vi "ConnectToAdaptorr02.vi"(1 "error in (no error)":errorcluster) -> (0 "error out":errorcluster, 2 "VISA resource name out":refnum<visa-resource-name>)   [LabVIEW 2011]
uses:
  <vilib>/Utility/error.llb/DialogType.ctl
  <vilib>/Instr/_visa.llb/VISA Configure Serial Port (Instr).vi
panel:
  out "message":string="AdaptTorr error!"
  in  "flow control":u16(ring) items=["None"=0, "XON/XOFF"=1, "RTS/CTS"=2, "DTR/DSR"=4]
  in  "stop bits":u16(ring)=20 items=["2"=10, "1.5"=15, "2.0"=20]
  in  "parity":u16(ring) items=["None", "Odd", "Even", "Mark", "Space"]
  in  "data bits":u16=8 min=5 max=8 step=1
  in  "VISA resource name":refnum<visa-resource-name>="COM8"
  in  "baud rate":u32=9600
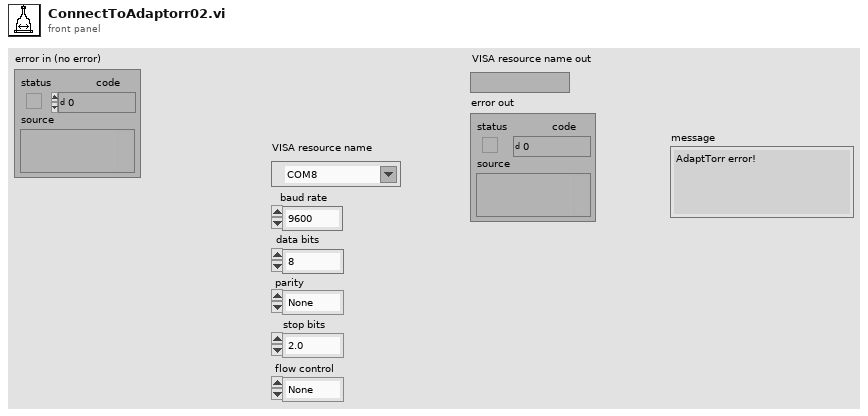
[diagram p1: front panel]
types:
  T1 = typedef "DialogType.ctl" = u16
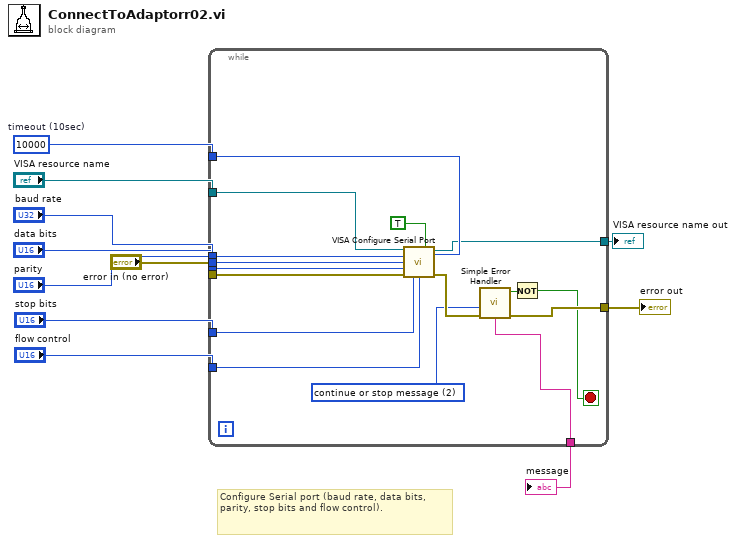
[diagram p0: block diagram]
diagram:
  w8 = u32 10000  # timeout (10sec)
  # "Configure Serial port (baud rate, data bits, parity, stop bits and flow control)."
  n1 = while {
    tunnel: "baud rate" -> [w27]
    tunnel: "VISA resource name" -> [w26]
    tunnel: "parity" -> [w25]
    tunnel: w8 -> [w24]
    tunnel: "stop bits" -> [w23]
    tunnel: "flow control" -> [w22]
    tunnel: "data bits" -> [w21]
    tunnel: [w20] -> w4
    tunnel: "error in (no error)" -> [w19]
    tunnel: [w18] -> w2
    tunnel: [w17] -> w1
    stop <- w16 stop-if-true
    w13 = T1 2 items=["no dialog", "OK message", "continue or stop message", "OK message + warnings", "continue/stop + warnings"] ("type of dialog (OK msg:1)")
    n2 = call-poly "VISA Configure Serial Port"("VISA resource name"=w26, "timeout (10sec)"=w24, "Enable Termination\nChar (T)"=TRUE ("Enable Termination\nChar (T)"), "baud rate (9600)"=w27, "data bits (8)"=w21, "parity (0:none)"=w25, "error in (no error)"=w19, "stop bits (10: 1 bit)"=w23, "flow control (0:none)"=w22) -> ("VISA resource name out"=w20:refnum<visa-resource-name>, "error out"=w14:errorcluster)  [unwired: 5 out]
    n3 = call <vilib>:"Simple Error Handler.vi"("type of dialog (OK msg:1)"=w13, "error in (no error)"=w14) -> ("error?"=w12:bool, "error out"=w18:errorcluster, "message"=w17:string)  [unwired: 3 in, 2 out]
    n4 = Not(x=w12) -> (.not. x?=w16:bool)
  }
  "VISA resource name out" <- w4
  "error out" <- w2
  "message" <- w1
